vi "Set Minimum Log Level.vi"(8 "error in (no error)":errorcluster, 10 "log level":T1, 11 "logger name":string) -> (0 "error out":errorcluster)   [LabVIEW 2018, in "GLog.lvlib" / "Registry.lvlib"]
uses:
  Registry.lvlib
  api/logger_class/Log Levels.ctl
  Registry Actions.ctl
  dependencies/Utilities/Utilities.lvlib
  api/logger_class/Logger.lvclass
panel:
  # "Connector Pane"
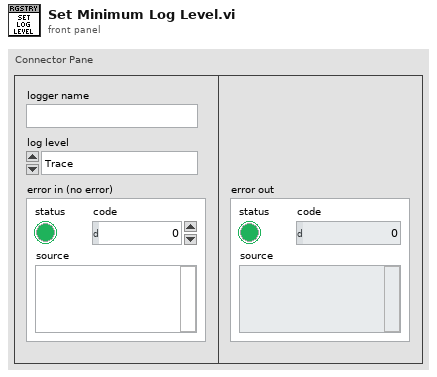
[diagram p1: front panel]
types:
  T1 = typedef "GLog.lvlib/Logger.lvclass/Log Levels.ctl" = enum16{"Trace", "Debug", "Info", "Warning", "Error", "Critical"}
  T2 = typedef "GLog.lvlib/Registry.lvlib/Registry Actions.ctl" = enum16{"Register", "Log", "Enable", "Enable All", "Disable", "Disable All", "Get Enable State", "Get Minimum Log Level", "Set Minimum Log Level", "Set All Minimum Log Level", "Get Logger Info", "Get All Logger Info", "List", "Unregister", "Unregister All", "Shutdown"}
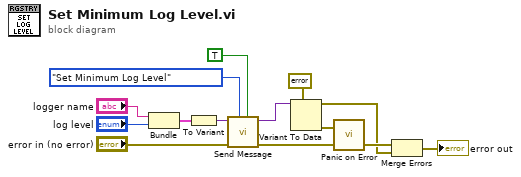
[diagram p0: block diagram]
diagram:
  n1 = Bundle("logger name"="logger name", "log level"="log level") -> (w4:cluster{"logger name":string, "log level":T1})  [unwired: 1 in]
  n2 = To Variant(anything=w4) -> (Variant=w10:variant)
  n3 = call "Send Message.vi"("return data? (F)"=TRUE, "action"=Registry_Actions."Set Minimum Log Level", "error in (no error)"="error in (no error)", "send data"=w10) -> ("error out"=w13:errorcluster, "return data"=w8:variant)  [unwired: 6 in]
  n4 = Variant To Data(type=errorcluster {"status"=FALSE, "code"=0, "source"=""} ("error out"), Variant=w8) -> (data=w2:errorcluster, error out=w7:errorcluster)  [unwired: 1 in]
  n5 = call "Panic on Error.vi"("error in (no error)"=w7) -> ()  [unwired: 3 in]
  n6 = Merge Errors(w13, w2) -> (→"error out":errorcluster)
